vi "Label Move.vi"(8 "error in (no error)":errorcluster, 9 "Owner Master Bounds Rect":T2, 10 "Label Position":T1, 11 "Label in":refnum<vi>) -> (0 "error out":errorcluster, 3 "dup Label":refnum<vi>)   [LabVIEW 2019, in "Builtins.lvlib"]
doc: "Moves the label to position specified.\n\nCreated by: Ryan Pacini"
uses:
  Builtins.lvlib
  Label Position.ctl
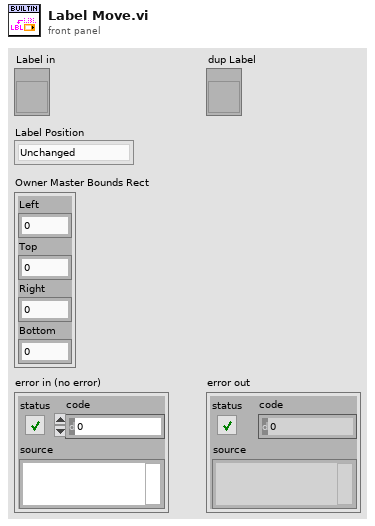
[diagram p1: front panel]
types:
  T1 = typedef "Builtins.lvlib/Label Position.ctl" = enum8{"Unchanged", "Top-left", "Top-middle", "Top-right", "Right-top", "Right-middle", "Right-bottom", "Bottom-right", "Bottom-middle", "Bottom-left", "Left-bottom", "Left-middle", "Left-top"}
  T2 = cluster{"Left":i16, "Top":i16, "Right":i16, "Bottom":i16}
  T3 = typedef "LVRectTypeDef.ctl" = cluster{"Left":i16, "Top":i16, "Right":i16, "Bottom":i16}
  T4 = typedef "LVPositionTypeDef.ctl" = cluster{"Left":i32, "Top":i32}
  T5 = cluster{"Left":i32, "Top":i32, "Right":i32, "Bottom":i32}
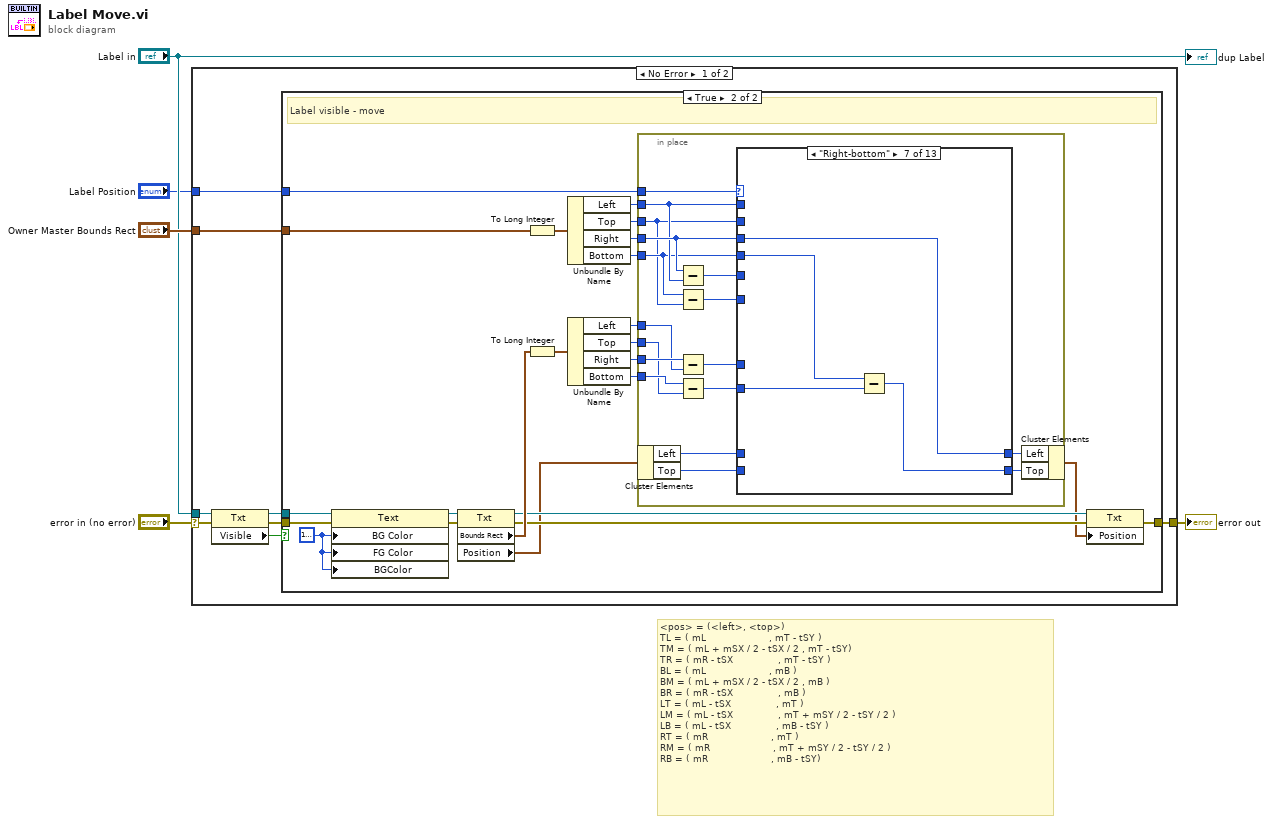
[diagram p0: block diagram]
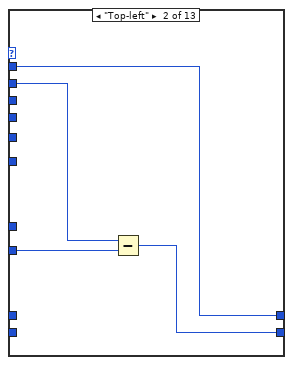
[diagram p4: hidden frame]
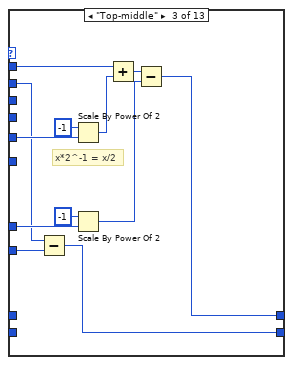
[diagram p5: hidden frame]
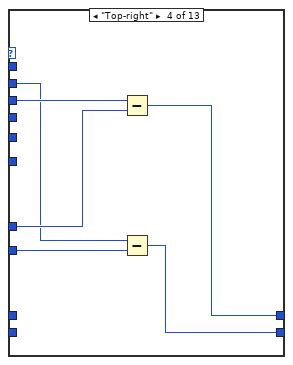
[diagram p6: hidden frame]
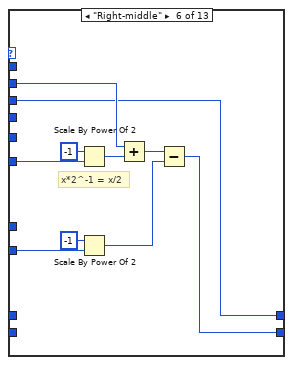
[diagram p8: hidden frame]
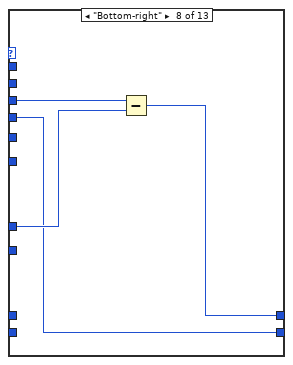
[diagram p9: hidden frame]
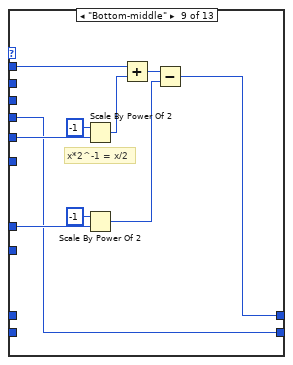
[diagram p10: hidden frame]
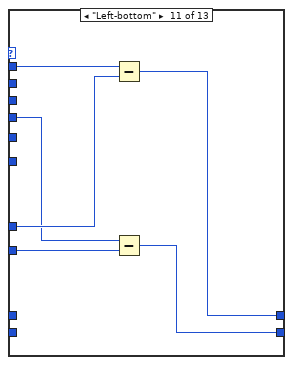
[diagram p12: hidden frame]
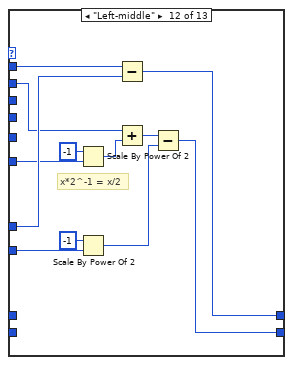
[diagram p13: hidden frame]
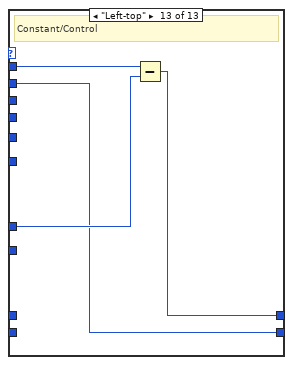
[diagram p14: hidden frame]
diagram:
  # "<pos> = (<left>, <top>)\nTL = ( mL                     , mT - tSY )\nTM = ( mL + mSX / 2 - tSX / 2 , mT - tSY)\nTR = ( mR - tSX               , mT - tSY )\nBL = ( mL                     , mB )\nBM = ( mL + mSX / 2 - tSX / 2 , mB )\nBR = ( mR - tSX               , mB )\nLT = ( mL - tSX               , mT )\nLM = ( mL - tSX               , mT + mSY / 2 - tSY / 2 )\nLB = ( mL - tSX               , mB - tSY )\nRT = ( mR                     , mT )\nRM = ( mR                     , mT + mSY / 2 - tSY / 2 )\nRB = ( mR                     , mB - tSY)"
  n1 = case shown="No Error" "error in (no error)" {
    selector: "error in (no error)" -> [w7 w133]
    tunnel: [w6 w133] -> w2
    tunnel: "Label in" -> [w8 _]
    tunnel: "Owner Master Bounds Rect" -> [w10 _]
    tunnel: "Label Position" -> [w9 _]
    frame No Error {
      n2 = property class="Txt"(reference=w8, error in=w7) -> (reference out=w13:refnum<vi>, error out=w11:errorcluster, "Visible"=w12:bool)
      n3 = case shown="True" w12 {
        tunnel: w11 -> [w14 w36]
        tunnel: w13 -> [_ w35]
        tunnel: [w14 w34] -> w6
        tunnel: w9 -> [_ w16]
        tunnel: w10 -> [_ w33]
        frame False {
          # "Label hidden - do nothing"
        }
        frame True {
          w37 = u32 16777216
          # "Label visible - move"
          n4 = property class="Text"(reference=w35, error in=w36, "BG Color"=w37, "FG Color"=w37, "BGColor"=w37) -> (reference out=w28:refnum<vi>, error out=w29:errorcluster)
          n5 = property class="Txt"(reference=w28, error in=w29) -> (reference out=w22:refnum<vi>, error out=w21:errorcluster, "Bounds Rect"=w27:T3, "Position"=w18:T4)
          n6 = To Long Integer(number=w33) -> (32bit integer=w19:T5)
          n7 = To Long Integer(number=w27) -> (32bit integer=w20:T5)
          n8 = Unbundle By Name(w19) -> ("Left"=w31:i32, "Top"=w32:i32, "Right"=w30:i32, "Bottom"=w15:i32)
          n9 = Unbundle By Name(w20) -> ("Left"=w26:i32, "Top"=w25:i32, "Right"=w24:i32, "Bottom"=w23:i32)
          n10 = in-place {
            in-place-border: w16 -> [w54]
            in-place-border: w32 -> [w38]
            in-place-border: w31 -> [w40]
            in-place-border: w30 -> [w41]
            in-place-border: w26 -> [w48]
            in-place-border: w25 -> [w45]
            in-place-border: w24 -> [w49]
            in-place-border: w23 -> [w46]
            in-place-border: w15 -> [w39]
            n11 = in-place-cluster #1(w18) -> ("Left"=w53:i32, "Top"=w52:i32)
            n12 = Subtract(x=w41, y=w40) -> (x-y=w42:i32)
            n13 = Subtract(x=w39, y=w38) -> (x-y=w43:i32)
            n14 = Subtract(x=w49, y=w48) -> (x-y=w47:i32)
            n15 = Subtract(x=w46, y=w45) -> (x-y=w44:i32)
            n16 = case shown="\"Right-bottom\"" w54 {
              tunnel: [w55 w57 w61 w73 w79 w82 w91 w95 w99 w109 w111 w118 w129] -> w50
              tunnel: [w56 w58 w64 w74 w80 w81 w92 w96 w106 w110 w112 w117 w130] -> w51
              tunnel: w38 -> [_ w60 w63 w76 w79 w86 _ _ _ _ _ w121 w129]
              tunnel: w40 -> [_ w58 w72 _ _ _ _ _ w108 w110 w116 w128 w132]
              tunnel: w41 -> [_ _ _ w78 w80 w81 w92 w98 _ _ _ _ _]
              tunnel: w53 -> [w56 _ _ _ _ _ _ _ _ _ _ _ _]
              tunnel: w52 -> [w55 _ _ _ _ _ _ _ _ _ _ _ _]
              tunnel: w39 -> [_ _ _ _ _ _ w94 w95 w99 w109 w113 _ _]
              tunnel: w47 -> [_ _ w71 w77 _ _ _ w97 w102 _ w115 w127 w131]
              tunnel: w44 -> [_ w59 w62 w75 _ w87 w93 _ _ _ w114 w122 _]
              tunnel: w42 -> [_ _ w68 _ _ _ _ _ w103 _ _ _ _]
              tunnel: w43 -> [_ _ _ _ _ w88 _ _ _ _ _ w123 _]
              frame "Unchanged" {
              }
              frame "Top-left" {
                n17 = Subtract(x=w60, y=w59) -> (x-y=w57:i32)
              }
              frame "Top-middle" {
                # "x*2^-1 = x/2"
                n18 = Subtract(x=w63, y=w62) -> (x-y=w61:i32)
                n19 = Scale By Power Of 2(n=i16 -1, x=w68) -> (x*2^n=w67:i32)
                n20 = Scale By Power Of 2(n=i16 -1, x=w71) -> (x*2^n=w65:i32)
                n21 = Add(x=w72, y=w67) -> (x+y=w66:i32)
                n22 = Subtract(x=w66, y=w65) -> (x-y=w64:i32)
              }
              frame "Top-right" {
                n23 = Subtract(x=w78, y=w77) -> (x-y=w74:i32)
                n24 = Subtract(x=w76, y=w75) -> (x-y=w73:i32)
              }
              frame "Right-top" {
                # "Indicator"
              }
              frame "Right-middle" {
                # "x*2^-1 = x/2"
                n25 = Scale By Power Of 2(n=i16 -1, x=w88) -> (x*2^n=w85:i32)
                n26 = Scale By Power Of 2(n=i16 -1, x=w87) -> (x*2^n=w83:i32)
                n27 = Add(x=w86, y=w85) -> (x+y=w84:i32)
                n28 = Subtract(x=w84, y=w83) -> (x-y=w82:i32)
              }
              frame "Right-bottom" {
                n29 = Subtract(x=w94, y=w93) -> (x-y=w91:i32)
              }
              frame "Bottom-right" {
                n30 = Subtract(x=w98, y=w97) -> (x-y=w96:i32)
              }
              frame "Bottom-middle" {
                # "x*2^-1 = x/2"
                n31 = Scale By Power Of 2(n=i16 -1, x=w103) -> (x*2^n=w101:i32)
                n32 = Scale By Power Of 2(n=i16 -1, x=w102) -> (x*2^n=w100:i32)
                n33 = Add(x=w108, y=w101) -> (x+y=w107:i32)
                n34 = Subtract(x=w107, y=w100) -> (x-y=w106:i32)
              }
              frame "Bottom-left" {
              }
              frame "Left-bottom" {
                n35 = Subtract(x=w116, y=w115) -> (x-y=w112:i32)
                n36 = Subtract(x=w113, y=w114) -> (x-y=w111:i32)
              }
              frame "Left-middle" {
                # "x*2^-1 = x/2"
                n37 = Scale By Power Of 2(n=i16 -1, x=w123) -> (x*2^n=w120:i32)
                n38 = Scale By Power Of 2(n=i16 -1, x=w122) -> (x*2^n=w119:i32)
                n39 = Subtract(x=w128, y=w127) -> (x-y=w117:i32)
                n40 = Add(x=w121, y=w120) -> (x+y=w126:i32)
                n41 = Subtract(x=w126, y=w119) -> (x-y=w118:i32)
              }
              frame "Left-top" {
                # "Constant/Control"
                n42 = Subtract(x=w132, y=w131) -> (x-y=w130:i32)
              }
            }
            n43 = in-place-cluster #1("Left"=w51, "Top"=w50) -> (w17:T4)
          }
          n44 = property class="Txt"(reference=w22, error in=w21, "Position"=w17) -> (error out=w34:errorcluster)  [unwired: 1 out]
        }
      }
    }
    frame Error {
    }
  }
  "error out" <- w2
  "dup Label" <- "Label in"
